vi "CRYMicrophone Calibration.vi"(5 "Hardware in":string="Hardware        \u0000\u0001\u0000\u0000\u0000\u0000\u0000\u0000\u0000\u0000\u0000\u0000\u0000\u0000\u0000\u0000\u0000\u0000\u0000\u0000\u0000\u0000\u0000\u0000\u0000\u0000\u0000\u0000\u0000\u0000\u0000\u0000\u0000\u0000\u0000\u0000\u0000\u0000\u0000\u0000\u0000\u0000\u0000\u0000\u0000\u0000\u0000\u0000\u0000\u0000\u0000\u0012Digital Audio Labs\u0000\u0000\u0000\u0000\u0001\u0001@\b\u0000\u0000\u0000\u0000\u0000\u0000@\b\u0000\u0000\u0000\u0000\u0000\u0000\u0000\u0000¬D\u0001\u0002?þáG®\u0014zá", 8 "Microphone":u16(ring)=3 items=["CRY 33x", "B&K Type 4133/4191", "B&K Type 4134/4192", "Other Microphones"], 9 "Calibrator":u16(ring)=3 items=["CRY 5611", "B&K Type 4231/4230", "B&K Type 4228/4220", "Other Calibrator"], 10 "Pre-Gain:":dbl caption="预增益" step=1.0 format="%.1p", 11 "Old Total Sens":dbl=0.011643847615413707 step=1.0 format="%.4f") -> (0 "Ref. Freq out":dbl=1000.0 caption="8Ìà¬üÈÓÂ", 1 "Completed":bool, 2 "Measured Sensitivity":dbl caption="测量灵敏度" step=1.0 format="%.2p", 3 "Total Sens":dbl=0.011643847615413707 format="%.4f")   [LabVIEW 2013]
uses:
  <vilib>/Analysis/4window.llb/windowTd.ctl
  CRYCal Global.vi
  Stimulus/SubVI/CRYTime global.vi
  <vilib>/Analysis/0measdsp.llb/Scaled Time Domain Window (DBL).vi
  <vilib>/Analysis/NI_AALPro.lvlib
panel:
  out "est frequency peak":dbl format="%0.4f"
  out "est power peak":dbl format="%_6f"
  in  "Calibrate":bool
  in  "Cancel":bool
  in  "Cal. Input:":dbl=94.0 caption="校准输入" step=1.0 format="%.2f"
  in  "Ref. Freq:":dbl=1000.0 caption="参考频率"
  in  "Save":bool
  out "dB re. 1V/Pa":dbl(slide)=-90.0 scale=-60.0..-10.0 scale format="%.1p"
  out "Sensitivity Test:":bool
  out "Calib_board":bool caption="校准器"
  out "Measurement":bool caption="测量传声器"
  # "dB"
  # "Hz"
  # "dB"
  # "dB re 1V/Pa"
  # "V/Pa"
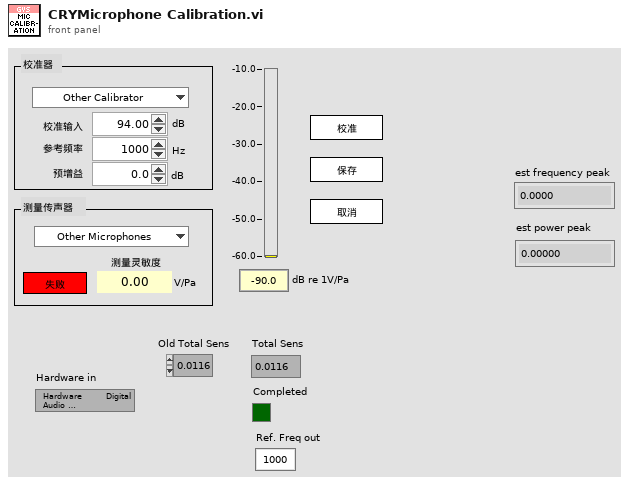
[diagram p1: front panel]
types:
  T1 = enum16{"OK", "Yes", "YesNo", "YesNoCancel", "ReplaceAppend"}
  T2 = typedef "NI_AALPro.lvlib/windowTd.ctl" = u32
  T3 = typedef "CRYWaveform Cluster Array.ctl" = T4[]
  T4 = typedef "CRYWaveform Cluster.ctl" = cluster{"Waveform":cluster{"X0":dbl, "dX":dbl, "Y":sgl[]}, "X data":u16, "Y data":u16, "Y axis":u16, "X unit":string, "Y unit":string, "Y dB ref":dbl, "display Y":bool, "display X":bool, "Overload?":bool, "Test Info":string, "Step No.":i32, "Name":string, "protected":bool, "Sqc history":string[], "Signal Channel ID":i32, "Plot Settings":cluster{"Color":u32, "Interpolation":u8, "Point Style":u8, "Line Style":u8, "Point Color":u32, "Line Width":u8, "Bar Plot Style":u8, "Fill To":i16}, "AutoProtect":bool}
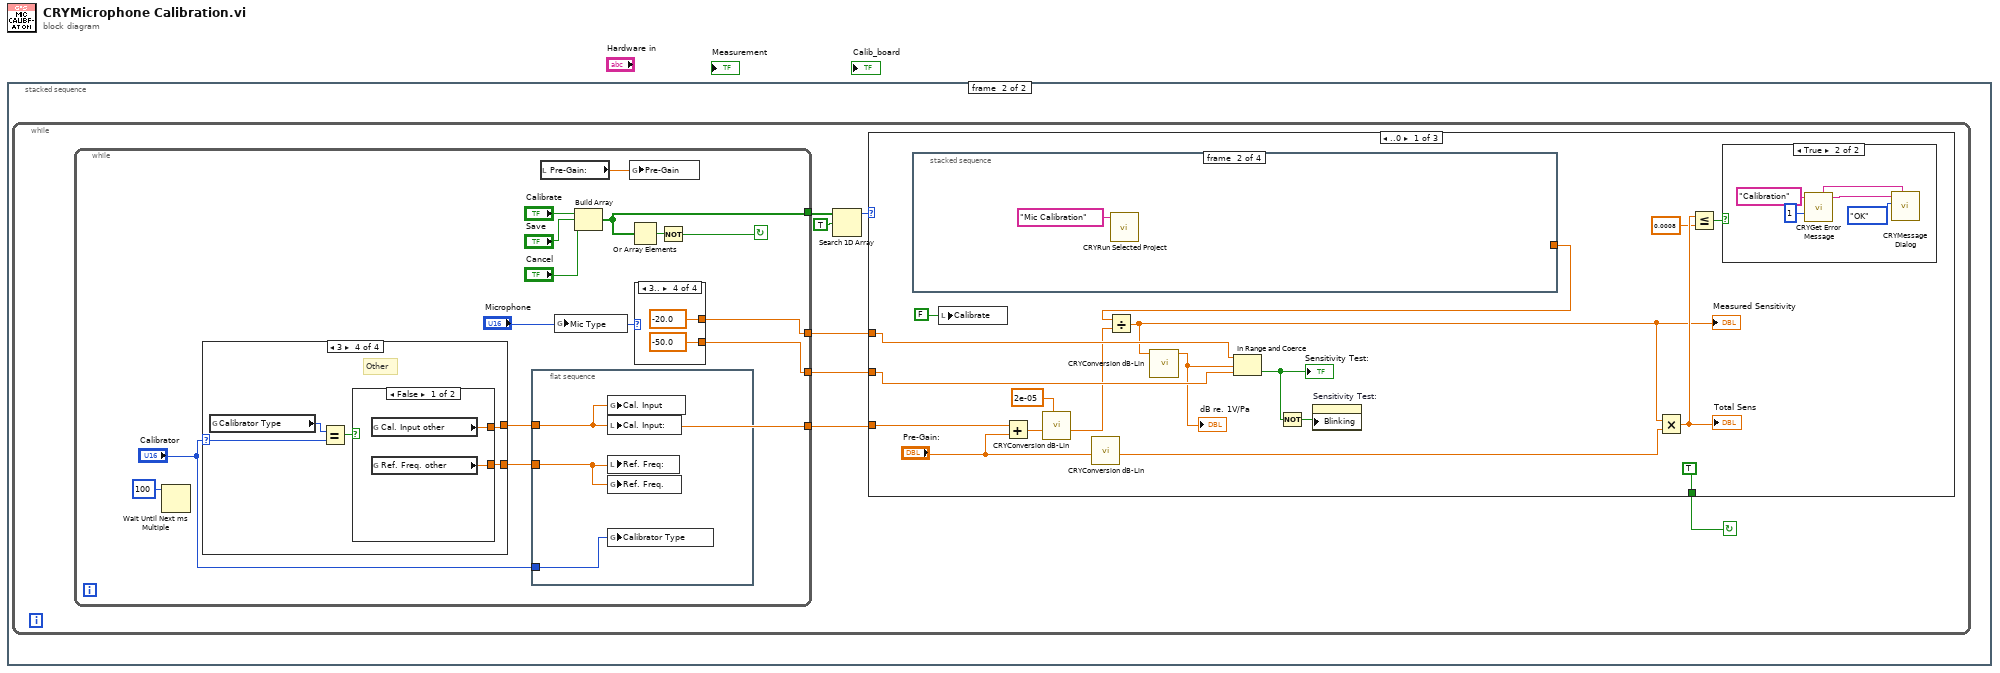
[diagram p0: block diagram]
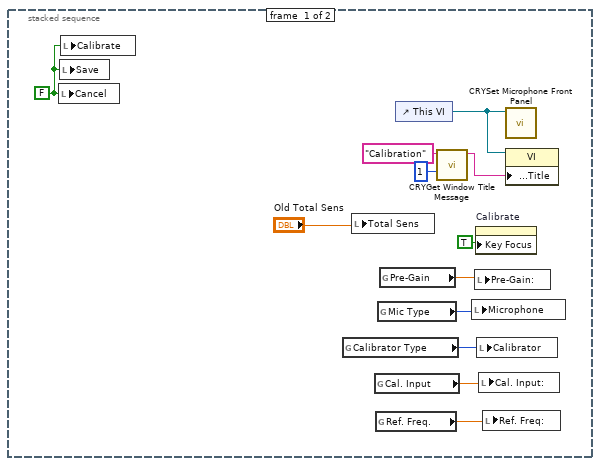
[diagram p2: hidden frame]
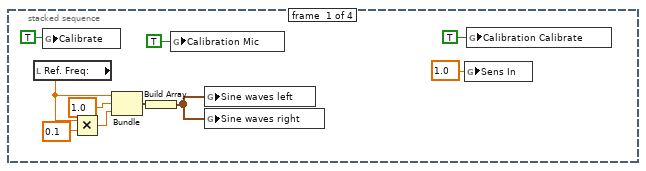
[diagram p4: hidden frame]
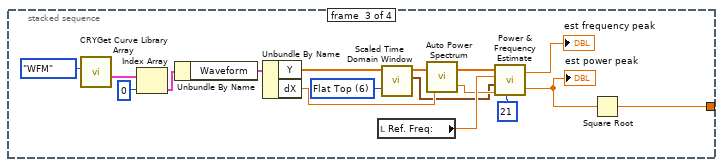
[diagram p5: hidden frame]
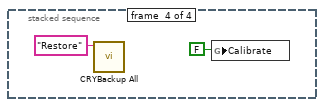
[diagram p6: hidden frame]
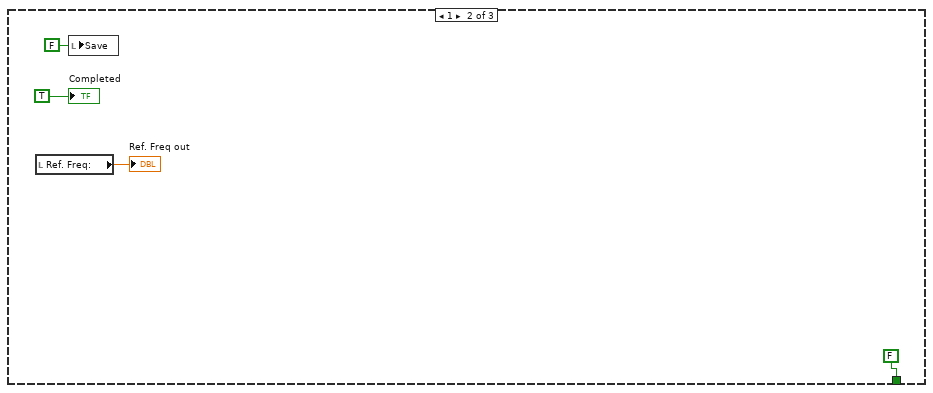
[diagram p7: hidden frame]
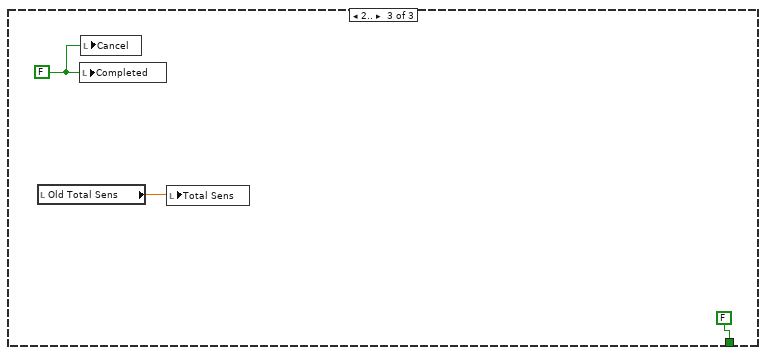
[diagram p8: hidden frame]
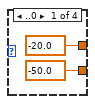
[diagram p9: hidden frame]
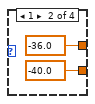
[diagram p10: hidden frame]
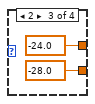
[diagram p11: hidden frame]
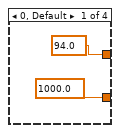
[diagram p12: hidden frame]
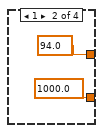
[diagram p13: hidden frame]
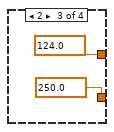
[diagram p14: hidden frame]
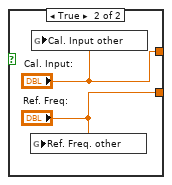
[diagram p15: hidden frame]
diagram:
  n1 = stacked-sequence {
    frame #0 {
      w1 = FALSE ("Cancel")
      n2 = local write "Cancel"(w1) -> ()
      n3 = local write "Save"(w1) -> ()
      n4 = local write "Calibrate"(w1) -> ()
      n5 = global read "CRYCal Global.vi" "Calibrator Type"() -> (w8:u16)
      n6 = local write "Total Sens"("Old Total Sens") -> ()
      n7 = global read "CRYCal Global.vi" "Cal. Input"() -> (w7:dbl)
      n8 = global read "CRYCal Global.vi" "Ref. Freq."() -> (w6:dbl)
      n9 = global read "CRYCal Global.vi" "Mic Type"() -> (w9:u16)
      n10 = global read "CRYCal Global.vi" "Pre-Gain"() -> (w10:dbl)
      n11 = control-ref of="This VI"() -> (w3:refnum<vi>)
      n12 = call "CRYGet Window Title Message.vi"("No"=1, "Kind"="Calibration") -> ("Multibyte String"=w2:string)  [unwired: 4 in, 5 out]
      n13 = local write "Microphone"(w9) -> ()
      n14 = local write "Pre-Gain:"(w10) -> ()
      n15 = property on="Calibrate" class="Bool (strict)"("Key Focus"=TRUE ("Write Attribute")) -> ()  [unwired: 2 in, 2 out]
      n16 = local write "Calibrator"(w8) -> ()
      n17 = local write "Cal. Input:"(w7) -> ()
      n18 = local write "Ref. Freq:"(w6) -> ()
      n19 = call "CRYSet Microphone Front Panel.vi"("Vi Ref"=w3) -> ()  [unwired: 11 in]
      n20 = property class="VI"(reference=w3, "Front Panel.Title"=w2) -> ()  [unwired: 1 in, 2 out]
    }
    frame #1 {
      n21 = while {
        stop <- w13 continue-if-true
        n22 = while {
          tunnel: [w88] -> w15
          tunnel: [w84] -> w19
          tunnel: [w92] -> w18
          tunnel: [w91] -> w17
          stop <- w80 continue-if-true
          n23 = Wait Until Next ms Multiple(millisecond multiple=100) -> ()  [unwired: 1 out]
          n24 = case shown="3" "Calibrator" {
            selector: "Calibrator" -> [_ _ _ w112]
            tunnel: [94.0 94.0 124.0 ("Cal. Input:") w115] -> w84
            tunnel: [1000.0 1000.0 250.0 ("Ref. Freq.:") w114] -> w82
            frame 0, Default {
            }
            frame 1 {
            }
            frame 2 {
            }
            frame 3 {
              # "Other"
              n25 = global read "CRYCal Global.vi" "Calibrator Type"() -> (w113:u16)
              n26 = Equal?(x=w113, y=w112) -> (x = y?=w111:bool)
              n27 = case shown="False" w111 {
                tunnel: [w117 "Cal. Input:"] -> w115
                tunnel: [w116 "Ref. Freq:"] -> w114
                frame False {
                  n28 = global read "CRYCal Global.vi" "Cal. Input other"() -> (w117:dbl)
                  n29 = global read "CRYCal Global.vi" "Ref. Freq. other"() -> (w116:dbl)
                }
                frame True {
                  n30 = global write "CRYCal Global.vi" "Ref. Freq. other"("Ref. Freq:") -> ()
                  n31 = global write "CRYCal Global.vi" "Cal. Input other"("Cal. Input:") -> ()
                }
              }
            }
          }
          n32 = flat-sequence {
            tunnel: w84 -> [w96]
            tunnel: "Calibrator" -> [w95]
            tunnel: w82 -> [w94]
            frame #0 {
              n33 = global write "CRYCal Global.vi" "Cal. Input"(w96) -> ()
              n34 = local write "Cal. Input:"(w96) -> ()
              n35 = local write "Ref. Freq:"(w94) -> ()
              n36 = global write "CRYCal Global.vi" "Ref. Freq."(w94) -> ()
              n37 = global write "CRYCal Global.vi" "Calibrator Type"(w95) -> ()
            }
          }
          n38 = local read "Pre-Gain:"() -> (w86:dbl)
          n39 = global write "CRYCal Global.vi" "Mic Type"("Microphone") -> ()
          n40 = Build Array("Calibrate", "Save", "Cancel") -> (w88:bool[])
          n41 = global write "CRYCal Global.vi" "Pre-Gain"(w86) -> ()
          n42 = Or Array Elements(Boolean array=w88) -> (logical OR=w81:bool)
          n43 = case shown="3.." "Microphone" {
            tunnel: [-20.0 -36.0 -24.0 -20.0] -> w92
            tunnel: [-50.0 -40.0 -28.0 -50.0] -> w91
            frame ..0 {
            }
            frame 1 {
            }
            frame 2 {
            }
            frame 3.. {
            }
          }
          n44 = Not(x=w81) -> (.not. x?=w80:bool)
        }
        n45 = Search 1D Array(1D array=w15, element=TRUE) -> (index of element=w14:i32)  [unwired: 1 out]
        n46 = case shown="..0" w14 {
          tunnel: [TRUE FALSE FALSE] -> w13
          tunnel: w19 -> [w36 _ _]
          tunnel: w18 -> [w35 _ _]
          tunnel: w17 -> [w34 _ _]
          frame ..0 {
            n47 = stacked-sequence {
              tunnel: [_ _ w54 _] -> w21
              frame #0 {
                n48 = local read "Ref. Freq:"() -> (w48:dbl)
                n49 = global write "CRYCal Global.vi" "Calibrate"(TRUE ("Calibrate")) -> ()
                n50 = Multiply(x=w48, y=0.1) -> (x*y=w51:dbl)
                n51 = Bundle("Ref. Freq:"=w48, "Sens In"=1.0, w51) -> (w52:cluster{"Ref. Freq:":dbl, "Sens In":dbl, dbl})  [unwired: 1 out]
                n52 = Build Array(w52) -> (w46:cluster{"Ref. Freq:":dbl, "Sens In":dbl, dbl}[])
                n53 = global write "CRYCal Global.vi" "Calibration Mic"(TRUE ("Calibration Mic")) -> ()
                n54 = global write "CRYTime global.vi" "Sine waves left"(w46) -> ()
                n55 = global write "CRYTime global.vi" "Sine waves right"(w46) -> ()
                n56 = global write "CRYCal Global.vi" "Sens In"(1.0 ("Sens In")) -> ()
                n57 = global write "CRYCal Global.vi" "Calibration Calibrate"(TRUE ("Calibration Calibrate")) -> ()
              }
              frame #1 {
                n58 = call "CRYRun Selected Project.vi"("sequence name"="Mic Calibration" ("Sequence")) -> ()  [unwired: 11 out]
              }
              frame #2 {
                w56 = T2 6 items=["Rectangle"=0, "Hanning"=1, "Hamming"=2, "Blackman-Harris"=3, "Exact Blackman"=4, "Blackman"=5, "Flat Top"=6, "4 Term B-Harris "=7, "7 Term B-Harris"=8, "Low Sidelobe"=9, "Blackman Nuttall"=11, "Triangle"=30, "Bartlett-Hanning"=31, "Bohman"=32, "Parzen"=33, "Welch"=34, "Kaiser"=60, "Dolph-Chebyshev"=61, "Gaussian"=62] ("window")
                n59 = call "CRYGet Curve Library Array.vi"("Type In"=enum16{"Curves", "Values", "Results", "WFM"}."WFM") -> ("Waveform Array"=w66:T3)  [unwired: 8 in, 2 out]
                n60 = Index Array(array=w66, index=0) -> (element=w69:T4)
                n61 = Unbundle By Name(w69) -> ("Waveform"=w68:cluster{"X0":dbl, "dX":dbl, "Y":sgl[]})
                n62 = Unbundle By Name(w68) -> ("Y"=w59:sgl[], "dX"=w65:dbl)
                n63 = local read "Ref. Freq:"() -> (w64:dbl)
                n64 = call-poly <vilib>:"Scaled Time Domain Window.vi"("window"=w56, "X"=w59) -> ("window properties"=w58:cluster{"eq noise BW":dbl, "coherent gain":dbl}, "Windowed X"=w57:dbl[])  [unwired: 7 in, 1 out]
                n65 = call <vilib>:"Auto Power Spectrum.vi"("dt"=w65, "Signal (V)"=w57) -> ("df"=w62:dbl, "Power Spectrum (V^2 rms)"=w61:dbl[])
                n66 = call <vilib>:"Power & Frequency Estimate.vi"("span"=21, "df"=w62, "window constants"=w58, "peak frequency (max)"=w64, "Power Spectrum (V^2 rms)"=w61) -> ("est power peak"=w55:dbl, "est frequency peak"=→"est frequency peak":dbl)  [unwired: 1 in]
                "est power peak" <- w55
                n67 = Square Root(x=w55) -> (sqrt(x)=w54:dbl)
              }
              frame #3 {
                n68 = call "CRYBackup All.vi"("sOption"="Restore") -> ()  [unwired: 11 in]
                n69 = global write "CRYCal Global.vi" "Calibrate"(FALSE ("Calibrate")) -> ()
              }
            }
            n70 = local write "Calibrate"(FALSE ("Cancel")) -> ()
            n71 = Add(x=w36, y="Pre-Gain:") -> (x+y=w24:dbl)
            n72 = call "CRYConversion dB-Lin.vi"("dB ref."=2e-05, "Log In"=w24) -> ("Lin Out"=w22:dbl)  [unwired: 4 in, 3 out]
            n73 = call "CRYConversion dB-Lin.vi"("Log In"="Pre-Gain:") -> ("Lin Out"=w25:dbl)  [unwired: 5 in, 3 out]
            n74 = Divide(x=w21, y=w22) -> (x/y=w20:dbl)
            "Measured Sensitivity" <- w20
            n75 = call "CRYConversion dB-Lin.vi"("Lin In"=w20) -> ("Log Out"=w28:dbl)  [unwired: 5 in, 3 out]
            "dB re. 1V/Pa" <- w28
            n76 = In Range and Coerce(upper limit=w35, x=w28, lower limit=w34) -> (In Range?=w29:bool)  [unwired: 1 out]
            "Sensitivity Test:" <- w29
            n77 = Not(x=w29) -> (.not. x?=w33:bool)
            n78 = property on="Sensitivity Test:" class="Bool (strict)"("Blinking"=w33) -> ()  [unwired: 2 in, 2 out]
            n79 = Multiply(x=w20, y=w25) -> (x*y=w31:dbl)
            "Total Sens" <- w31
            n80 = Less Or Equal?(x=w31, y=0.0008) -> (x <= y?=w32:bool)
            n81 = case shown="True" w32 {
              frame False {
              }
              frame True {
                n82 = call "CRYGet Error Message.vi"("Error No"=1, "Kind"="Calibration") -> ("Message"=w38:string, "Window Title"=w39:string)  [unwired: 4 in, 4 out]
                n83 = call "CRYMessage Dialog.vi"("Window Title"=w39, "YesNoCancel"=T1."OK", "Message Content"=w38) -> ()  [unwired: 7 in, 2 out]
              }
            }
          }
          frame 1 {
            n84 = local read "Ref. Freq:"() -> (→"Ref. Freq out":dbl)
            n85 = local write "Save"(FALSE ("Save")) -> ()
            "Completed" <- TRUE ("Completed")
          }
          frame 2.. {
            w77 = FALSE ("Completed")
            n86 = local read "Old Total Sens"() -> (w78:dbl)
            n87 = local write "Completed"(w77) -> ()
            n88 = local write "Cancel"(w77) -> ()
            n89 = local write "Total Sens"(w78) -> ()
          }
        }
      }
    }
  }
